vi "MALT DeviceReqW2PCreate.vi"(6 "Param2":i32=-1, 7 "Cmd":string, 8 "error in":errorcluster, 9 "Param1":i32, 10 "Address":i32, 11 "CardType":T1=enum."MALT132") -> (0 "error out":errorcluster, 3 "Request":string="@03:00:SET#ONE:00")   [LabVIEW 2018, in "AltonTech MALT200817.lvlib"]
uses:
  <instrlib>/AltonTech MALT/AltonTech MALT200817.lvlib
  <instrlib>/AltonTech MALT/Public/Types/MALT Family Codes.ctl
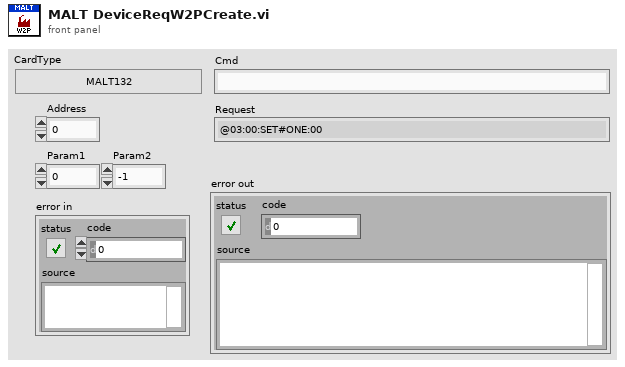
[diagram p1: front panel]
types:
  T1 = typedef "AltonTech MALT200817.lvlib/MALT Family Codes.ctl" = enum32{"-", "YAV90832", "YAV904X8", "MALT132", "YAV91616", "MALT16PIN", "YAV90096", "YAV90HVT", "YAV90CLR", "YAV90128", "YAV90PNE", "YAVCANCON", "YAV91775", "YAV90XXX", "YAV90MMU", "H730050", "H710060", "H710061", "YAV90304", "MMI", "YAV90060", "MALT160T", "YAV90059", "Not Defined"}
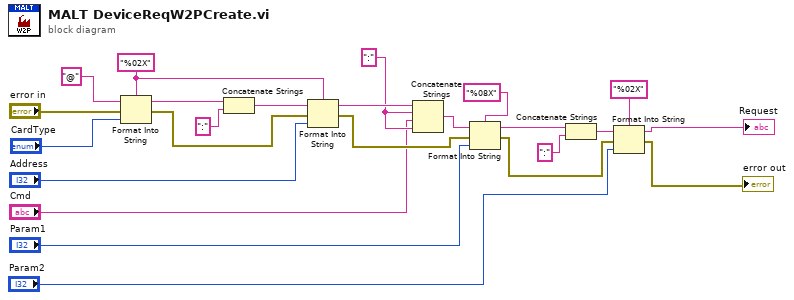
[diagram p0: block diagram]
diagram:
  w13 = ":" ("resulting string")
  w5 = "%02X" ("format string")
  n1 = Format Into String(format string=w5, initial string="@", error in="error in", "CardType") -> (resulting string=w23:string, error out=w18:errorcluster)
  n2 = Concatenate Strings(w23, ":" ("string")) -> (w21:string)
  n3 = Format Into String(format string=w5, initial string=w21, error in=w18, "Address") -> (resulting string=w19:string, error out=w16:errorcluster)
  n4 = Concatenate Strings(w19, w13, "Cmd", w13) -> (w17:string)
  n5 = Format Into String(format string="%08X", initial string=w17, error in=w16, "Param1") -> (resulting string=w8:string, error out=w7:errorcluster)
  n6 = Concatenate Strings(w8, ":" ("string")) -> (w2:string)
  n7 = Format Into String(format string="%02X", initial string=w2, error in=w7, "Param2") -> (resulting string=→"Request":string, error out=→"error out":errorcluster)
